vi "FixMgiMonitoredActor.vi"   [LabVIEW 2020]
uses:
  <vilib>/Utility/EditLVLibs/Edit LVLibs.lvlib
types:
  T1 = enum32{"Invalid", "Standard", "Closed", "Hidden", "Minimized", "Maximized"}
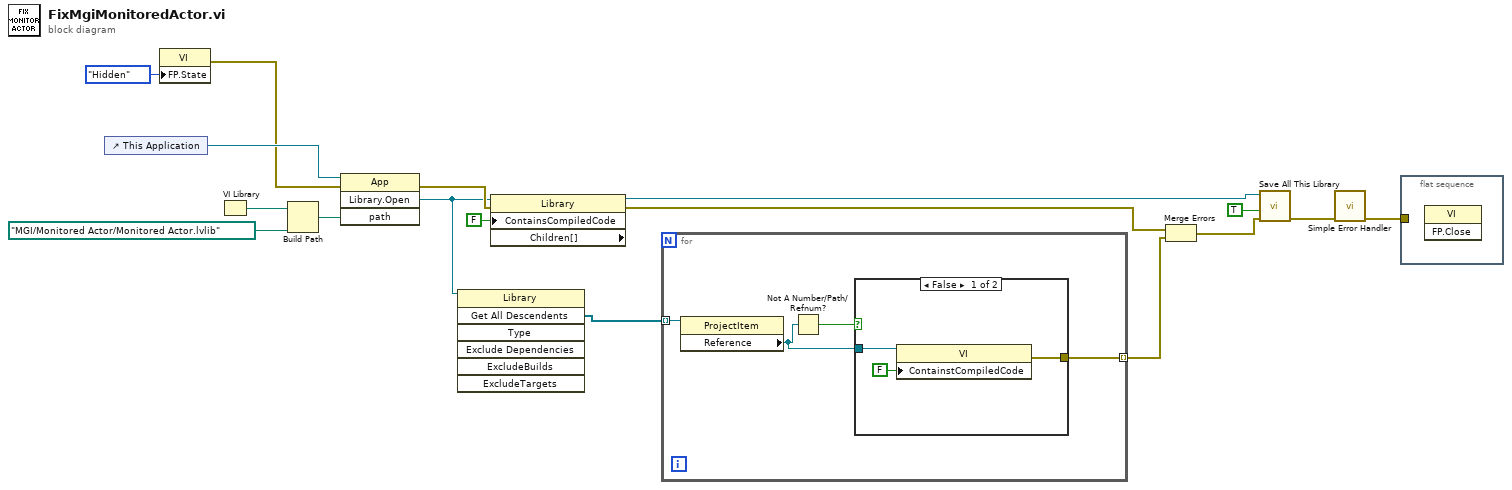
[diagram p0: block diagram]
diagram:
  n1 = control-ref of="This Application"() -> (w13:refnum<vi>)
  n2 = property class="VI"("FP.State"=T1."Hidden" ("Front Panel Window:State")) -> (error out=w1:errorcluster)  [unwired: 2 in, 1 out]
  n3 = VI Library() -> (path=w10:path)
  n4 = Build Path(base path=w10, name or relative path=path "MGI/Monitored Actor/Monitored Actor.lvlib") -> (appended path=w12:path)
  n5 = invoke class="App" method="Library.Open"(reference=w13, error in=w1, "path"=w12) -> (error out=w17:errorcluster, "Open Library"=w4:refnum<vi>)  [unwired: 1 in, 2 out]
  n6 = invoke class="Library" method="Get All Descendents"(reference=w4) -> ("All Descendents"=w3:refnum<vi>[])  [unwired: 6 in, 6 out]
  n7 = property class="Library"(reference=w4, error in=w17, "ContainsCompiledCode"=FALSE ("Contains Compiled Code")) -> (reference out=w8:refnum<vi>, error out=w15:errorcluster, "Children[]"=w6:refnum<vi>[])
  n8 = for {
    tunnel: [w22] -> w5 mode=indexing
    tunnel: w3 -> [w19] mode=indexing
    n9 = property class="ProjectItem"(reference=w19) -> ("Reference"=w20:refnum<vi>)  [unwired: 1 in, 2 out]
    n10 = Not A Number/Path/Refnum?(number/path/refnum=w20) -> (NaN/Path/Refnum?=w21:bool)
    n11 = case shown="False" w21 {
      tunnel: w20 -> [w23 _]
      tunnel: [w25 _] -> w22
      frame False {
        n12 = property class="VI"(reference=w23, "ContainstCompiledCode"=FALSE ("Contains Compiled Code")) -> (error out=w25:errorcluster)  [unwired: 1 in, 1 out]
      }
      frame True {
      }
    }
  }
  n13 = Merge Errors(w15, w5) -> (w14:errorcluster)
  n14 = call <vilib>:"Save All This Library.vi"("error in (no error)"=w14, "Save Only Modified VIs and Libraries? (F)"=TRUE, "Library in"=w8) -> ("error out"=w16:errorcluster)  [unwired: 7 in, 1 out]
  n15 = call <vilib>:"Simple Error Handler.vi"("error in (no error)"=w16) -> ("error out"=w18:errorcluster)  [unwired: 4 in, 4 out]
  n16 = flat-sequence {
    tunnel: w18 -> [_]
    frame #0 {
      n17 = invoke class="VI" method="FP.Close"() -> ()  [unwired: 3 in, 3 out]
    }
  }
